vi "Open4Motors.vi"(6 "Invert":bool, 7 "Control Mode":T7, 8 "Rear Left Device Number":u8, 9 "Front Left Device Number":u8, 10 "Rear Right Device Number":u8, 11 "Front Right Device Number":u8) -> (1 "Left Motor":T1={"DeviceStatus"={"status"=FALSE, "code"=0, "source"=""}, "Type"=enum."PWM", "PWM"={"PWM Channel"=enum."Invalid", "DeadBand"={"Name"="", "maxPositivePwm"=0, "minPositivePwm"=0, "centerPwm"=0, "maxNegativePwm"=0, "minNegativePwm"=0, "angularRange"=0}}, "CAN"={"Device Number"=0, "Control Mode"=enum."Percent VBus", "Semaphore"=refnum, "Max Vout"=12.0, "TalonSRX Control Mode"=enum."Percent VBus"}, "Invert"=FALSE}, 2 "Right Motor":T1={"DeviceStatus"={"status"=FALSE, "code"=0, "source"=""}, "Type"=enum."PWM", "PWM"={"PWM Channel"=enum."Invalid", "DeadBand"={"Name"="", "maxPositivePwm"=0, "minPositivePwm"=0, "centerPwm"=0, "maxNegativePwm"=0, "minNegativePwm"=0, "angularRange"=0}}, "CAN"={"Device Number"=0, "Control Mode"=enum."Percent VBus", "Semaphore"=refnum, "Max Vout"=12.0, "TalonSRX Control Mode"=enum."Percent VBus"}, "Invert"=FALSE})   [LabVIEW 2015]
uses:
  <vilib>/Rock Robotics/WPI/CAN/TalonSRX/WPI_CANTalonSRX_APIControlMode.ctl
  <vilib>/Rock Robotics/WPI/MotorControl/WPI_MotorControlDeviceRef.ctl
  <vilib>/Rock Robotics/WPI/MotorControl/WPI_MotorControlType.ctl
  <vilib>/Rock Robotics/SystemInterfaces/DIO/FPGA_DIOPWMChannel.ctl
  <vilib>/Rock Robotics/WPI/PWM/WPI_PWMDeadband.ctl
  <vilib>/Rock Robotics/WPI/CAN/Jaguar/SubVIs/WPI_CANJaguar_ControlMode.ctl
  <vilib>/Rock Robotics/WPI/MotorControl/WPI_MotorControlOpenCANTalonSRX.vi
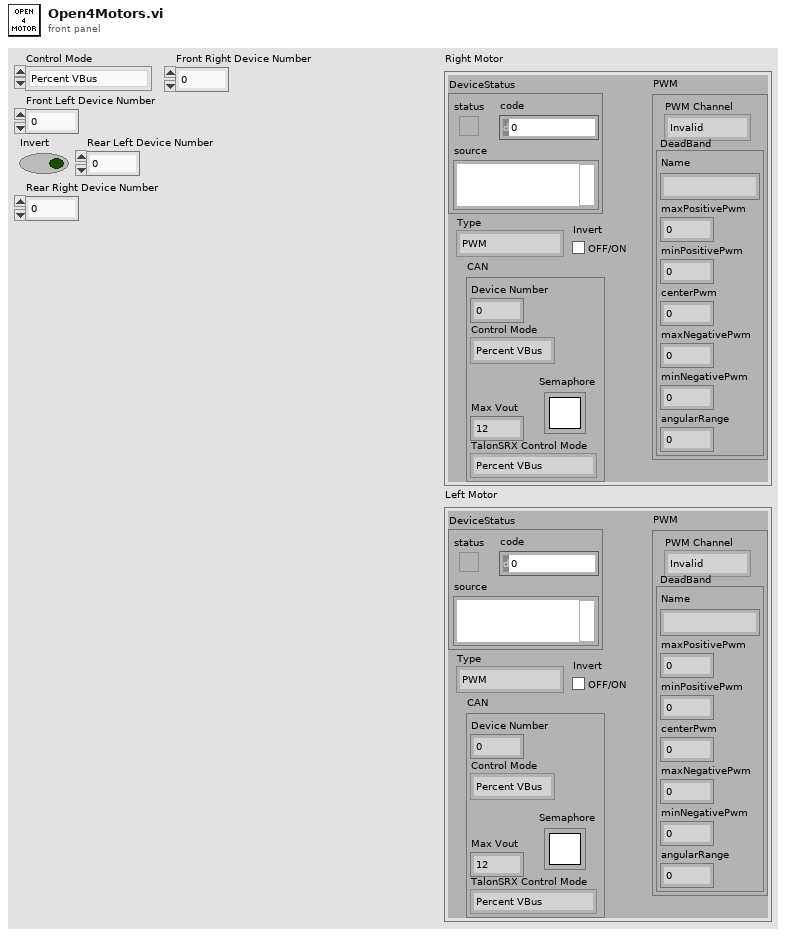
[diagram p1: front panel]
types:
  T1 = typedef "WPI_MotorControlDeviceRef.ctl" = cluster{"DeviceStatus":errorcluster, "Type":T2, "PWM":cluster{"PWM Channel":T3, "DeadBand":T4}, "CAN":cluster{"Device Number":u8, "Control Mode":T5, "Semaphore":T6, "Max Vout":dbl, "TalonSRX Control Mode":T7}, "Invert":bool}
  T2 = typedef "WPI_MotorControlType.ctl" = enum16{"PWM", "CAN", "CANTalonSRX"}
  T3 = typedef "FPGA_DIOPWMChannel.ctl" = enum8{"PWM 0", "PWM 1", "PWM 2", "PWM 3", "PWM 4", "PWM 5", "PWM 6", "PWM 7", "PWM 8", "PWM 9", "PWM MXP 0", "PWM MXP 1", "PWM MXP 2", "PWM MXP 3", "PWM MXP 4", "PWM MXP 5", "PWM MXP 6", "PWM MXP 7", "PWM MXP 8", "PWM MXP 9", "Invalid"}
  T4 = typedef "WPI_PWMDeadband.ctl" = cluster{"Name":string, "maxPositivePwm":i32, "minPositivePwm":i32, "centerPwm":i32, "maxNegativePwm":i32, "minNegativePwm":i32, "angularRange":u16}
  T5 = typedef "WPI_CANJaguar_ControlMode.ctl" = enum8{"Percent VBus", "Current", "Speed", "Position", "Voltage"}
  T6 = typedef "Semaphore RefNum" = refnum<k1>
  T7 = typedef "WPI_CANTalonSRX_APIControlMode.ctl" = enum8{"Percent VBus", "Speed", "Position", "Slave", "Unchanged / Invalid", "Voltage Compensation", "Current", "Motion Profile"}
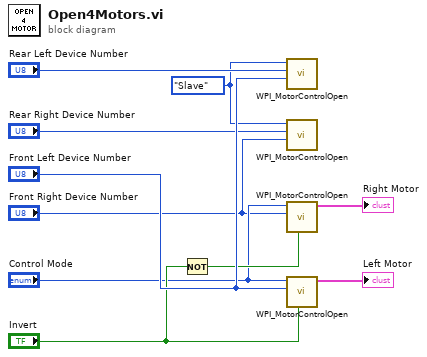
[diagram p0: block diagram]
diagram:
  w4 = WPI_CANTalonSRX_APIControlMode."Slave" ("Control Mode")
  n1 = Not(x="Invert") -> (.not. x?=w9:bool)
  n2 = call-poly <vilib>:"WPI_MotorControlOpen.vi"("Master Device Number"="Front Left Device Number", "Device Number"="Rear Left Device Number", "Control Mode"=w4) -> ()  [unwired: 2 in, 7 out]
  n3 = call-poly <vilib>:"WPI_MotorControlOpen.vi"("Master Device Number"="Front Right Device Number", "Device Number"="Rear Right Device Number", "Control Mode"=w4) -> ()  [unwired: 2 in, 7 out]
  n4 = call-poly <vilib>:"WPI_MotorControlOpen.vi"("Invert"=w9, "Device Number"="Front Right Device Number", "Control Mode"="Control Mode") -> ("MotorControlDeviceRef"=→"Right Motor":T1)  [unwired: 2 in, 6 out]
  n5 = call-poly <vilib>:"WPI_MotorControlOpen.vi"("Invert"="Invert", "Device Number"="Front Left Device Number", "Control Mode"="Control Mode") -> ("MotorControlDeviceRef"=→"Left Motor":T1)  [unwired: 2 in, 6 out]
